vi "pointerToObj.vi"(10 "stringIn":string) -> (2 "objOut":refnum<class>)   [LabVIEW 2009]
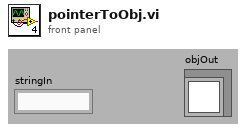
[diagram p1: front panel]
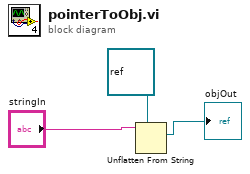
[diagram p0: block diagram]
diagram:
  n1 = Unflatten From String(type=refnum<class> refnum ("objOut"), binary string="stringIn") -> (value=→"objOut":refnum<class>)  [unwired: 3 in, 2 out]
